vi "PositionCount.vi"(0 "A":bool, 1 "ReversePolarity":bool, 5 "B":bool, 7 "Z":bool, 9 "reset":bool) -> (4 "AbsPosition":i32, 6 "RevPosition":i32, 15 "CW_direction":bool)   [LabVIEW 2015, in "QuadEnc.lvlib"]
uses:
  QuadEnc.lvlib
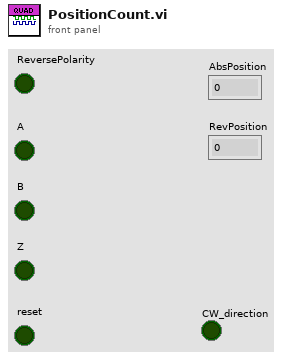
[diagram p1: front panel]
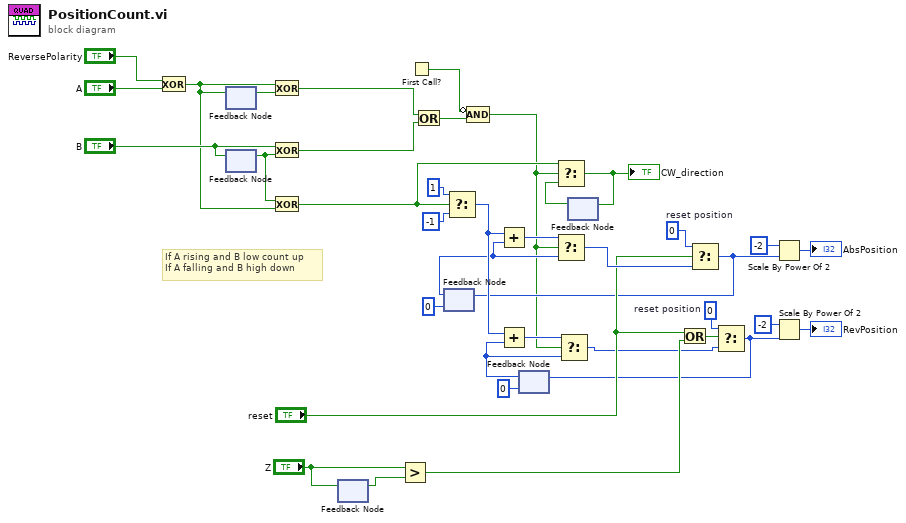
[diagram p0: block diagram]
diagram:
  w13 = 0  # reset position
  w21 = 0  # reset position
  # "If A rising and B low count up\nIf A falling and B high down"
  n1 = Exclusive Or(1:"A", 2:"ReversePolarity") -> (0:w32:bool)
  n2 = feedback #1() -> (w36:bool)  [unwired: 1 out]
  n3 = feedback-in #1(w32) -> ()
  n4 = feedback #2() -> (w31:bool)  [unwired: 1 out]
  n5 = feedback-in #2("B") -> ()
  n6 = Exclusive Or(1:w36, 2:w32) -> (0:w34:bool)
  n7 = Exclusive Or(1:w31, 2:"B") -> (0:w33:bool)
  n8 = Exclusive Or(1:w32, 2:w31) -> (0:w27:bool)
  n9 = feedback-in #3("Z") -> ()
  n10 = feedback #3() -> (w15:bool)  [unwired: 1 in]
  n11 = Greater?(x="Z", y=w15) -> (0:w11:bool)
  n12 = First Call?() -> (First Call?: T/F=w2:bool)
  n13 = Or(x=w34, y=w33) -> (x .or. y?=w3:bool)
  n14 = feedback #4(0) -> (w20:i32)
  n15 = Select(t=1, s=w27, f=-1) -> (s? t:f=w24:i32)
  n16 = Compound Arithmetic op=AND(invert w2, w3) -> (w1:bool)
  n17 = Add(x=w24, y=w20) -> (x+y=w28:i32)
  n18 = feedback #5(0) -> (w22:i32)
  n19 = Add(x=w24, y=w22) -> (x+y=w23:i32)
  n20 = Select(t=w28, s=w1, f=w20) -> (s? t:f=w17:i32)
  n21 = Select(t=w23, s=w1, f=w22) -> (s? t:f=w10:i32)
  n22 = feedback #6() -> (w25:bool)  [unwired: 1 out]
  n23 = Select(t=w27, s=w1, f=w25) -> (s? t:f=w26:bool)
  "CW_direction" <- w26
  n24 = feedback-in #6(w26) -> ()
  n25 = Or(x="reset", y=w11) -> (x .or. y?=w14:bool)
  n26 = Select(t=w21, s="reset", f=w17) -> (s? t:f=w9:i32)
  n27 = feedback-in #4(w9) -> ()
  n28 = Select(t=w13, s=w14, f=w10) -> (s? t:f=w4:i32)
  n29 = feedback-in #5(w4) -> ()
  n30 = Scale By Power Of 2(n=i16 -2, x=w9) -> (x*2^n=→"AbsPosition":i32)
  n31 = Scale By Power Of 2(n=i16 -2, x=w4) -> (x*2^n=→"RevPosition":i32)
